vi "PowerON.vi"(8 "error in (no error)":errorcluster, 11 "RoomLight in":refnum<class "RoomLight.lvclass">) -> (0 "error out":errorcluster, 2 "Message":string, 3 "RoomLight out":refnum<class "RoomLight.lvclass">)   [LabVIEW 2013, in "RoomLight.lvclass"]
uses:
  RoomLight.lvclass
  RoomLight.lvclass/RoomLight.ctl
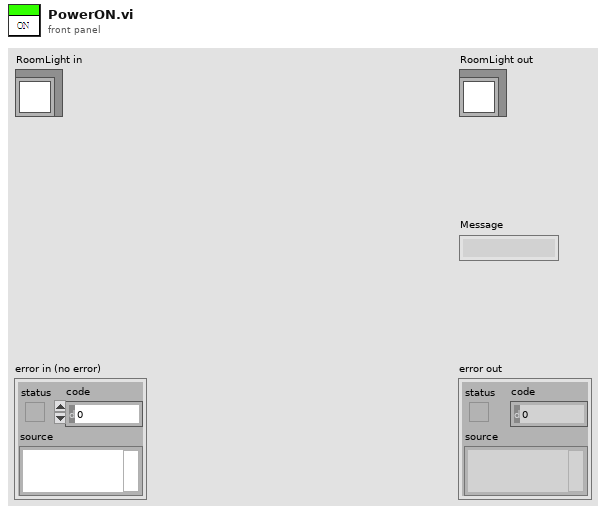
[diagram p1: front panel]
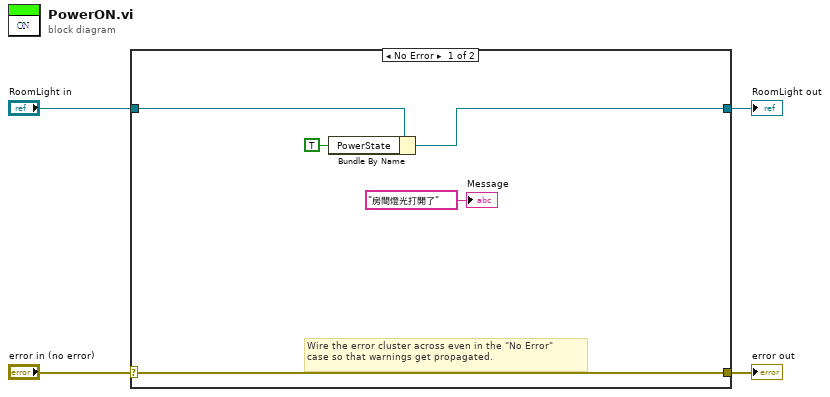
[diagram p0: block diagram]
diagram:
  n1 = case shown="No Error" "error in (no error)" {
    selector: "error in (no error)" -> [w9 w11]
    tunnel: [w9 w11] -> w3
    tunnel: [w6 w10] -> w1
    tunnel: "RoomLight in" -> [w7 w10]
    frame No Error {
      # "Wire the error cluster across even in the \"No Error\"\ncase so that warnings get propagated."
      n2 = Bundle By Name(cluster=w7, "PowerState"=TRUE) -> (w6:refnum<class "RoomLight.lvclass">)
      "Message" <- "房間燈光打開了" ("Message")
    }
    frame Error {
    }
  }
  "error out" <- w3
  "RoomLight out" <- w1
